vi "Send Voltage.vi"(8 "error in":errorcluster, 11 "6700C in":refnum<class "6700C.lvclass">) -> (0 "error out":errorcluster, 3 "6700C out":refnum<class "6700C.lvclass">)   [LabVIEW 2019, in "6700C.lvlib" / "6700C.lvclass"]
uses:
  Library/6700C.lvclass
  C:/Users/Public/Documents/Development/builds/Instruments/PowerSupply.lvlibp/Library/PowerSupply.lvclass
  Library/6700C.lvclass/6700C.ctl
  Accessors/Read Local Resource.vi
  Accessors/Write Local Resource.vi
  builds/Instruments/PowerSupply.lvlibp/Accessors/Read Active Channel.vi
  <instrlib>/Agilent N6700 Series/Agilent N6700 Series.lvlib
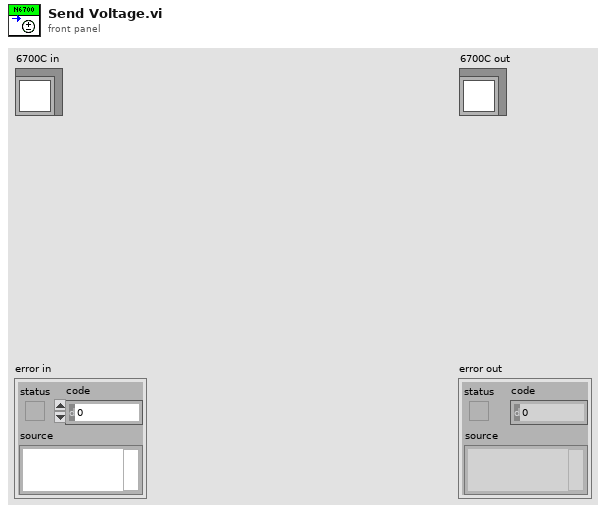
[diagram p1: front panel]
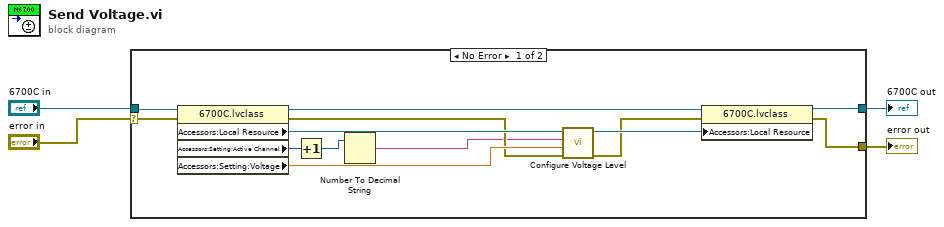
[diagram p0: block diagram]
diagram:
  n1 = case shown="No Error" "error in" {
    selector: "error in" -> [w14 w19]
    tunnel: [w15 w19] -> w4
    tunnel: [w16 w18] -> w3
    tunnel: "6700C in" -> [w17 w18]
    frame No Error {
      n2 = property class="6700C.lvclass"(reference=w17, error in=w14) -> (reference out=w10:refnum<class "6700C.lvclass">, error out=w8:errorcluster, "Accessors:Local Resource"=w11:refnum<visa-resource-name>, "Accessors:Setting:Active Channel"=w7:u32, "Accessors:Setting:Voltage"=w9:dbl)
      n3 = Increment(x=w7) -> (x+1=w5:u32)
      n4 = Number To Decimal String(number=w5) -> (decimal integer string=w6:string)  [unwired: 1 in]
      n5 = call <instrlib>:"Configure Voltage Level.vi"("error in (no error)"=w8, "Level  (0.0 volts)"=w9, "Channel Name (1)"=w6, "VISA resource name"=w11) -> ("error out"=w12:errorcluster, "VISA resource name out"=w13:refnum<visa-resource-name>)  [unwired: 6 in]
      n6 = property class="6700C.lvclass"(reference=w10, error in=w12, "Accessors:Local Resource"=w13) -> (reference out=w16:refnum<class "6700C.lvclass">, error out=w15:errorcluster)
    }
    frame Error {
    }
  }
  "error out" <- w4
  "6700C out" <- w3
